vi "NT Update Persistence.vi"(8 "error in":errorcluster, 10 "Persistence":bool=TRUE, 11 "Name":string="Numeric") -> (0 "error out":errorcluster)   [LabVIEW 2017]
doc: "Update the persistence setting for the variable."
uses:
  <vilib>/Rock Robotics/Network Tables/Create Actual Table Name.vi
  <vilib>/Rock Robotics/Network Tables/Table Manager.vi
  <vilib>/Rock Robotics/Network Tables/NT Globals.vi
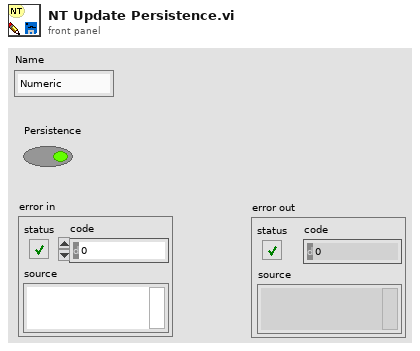
[diagram p1: front panel]
types:
  T1 = enum16{"Add", "Remove", "Clear", "Init", "Retrieve"}
  T2 = enum16{"Update Field", "Read Field", "Assign Field", "Remove All", "Set Persistence", "Clear Persistence"}
  T3 = typedef "Field ID.ctl" = i32
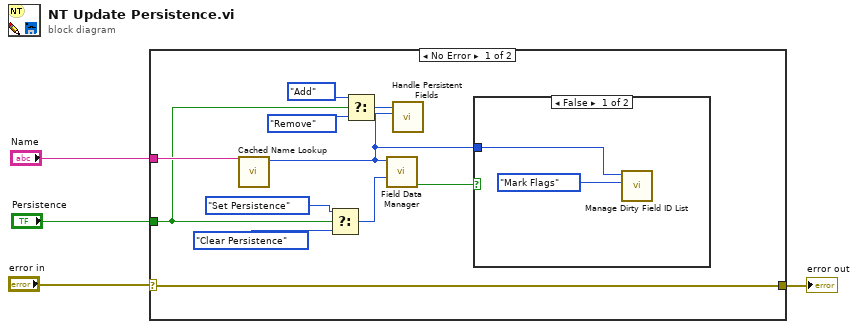
[diagram p0: block diagram]
diagram:
  n1 = case shown="No Error" "error in" {
    selector: "error in" -> [w15 w18]
    tunnel: "Persistence" -> [w8 _]
    tunnel: "Name" -> [w14 _]
    tunnel: [w15 w18] -> w2
    frame No Error {
      n2 = call <vilib>:"Cached Name Lookup.vi"("Name"=w14) -> ("Entry ID"=w5:T3)  [unwired: 8 in, 2 out]
      n3 = Select(t=T2."Set Persistence" ("Operation"), s=w8, f=T2."Clear Persistence" ("Operation")) -> (s? t:f=w11:T2)
      n4 = Select(t=T1."Add" ("Operation"), s=w8, f=T1."Remove" ("Operation")) -> (s? t:f=w7:T1)
      n5 = call <vilib>:"Field Data Manager.vi"("Operation"=w11, "Field ID"=w5) -> ("Equal"=w6:bool)  [unwired: 8 in, 1 out]
      n6 = call <vilib>:"Handle Persistent Fields.vi"("Field ID"=w5, "Operation"=w7) -> ()  [unwired: 9 in, 1 out]
      n7 = case shown="False" w6 {
        tunnel: w5 -> [w16 _]
        frame False {
          n8 = call <vilib>:"Manage Dirty Field ID List.vi"("Operation"=enum16{"Mark", "Retrieve/Clear", "Mark Flags"}."Mark Flags", "Field ID"=w16) -> ()  [unwired: 8 in, 2 out]
        }
        frame True {
        }
      }
    }
    frame Error {
    }
  }
  "error out" <- w2
